vi "Affichage PokaenDex 1P.vi"() -> ()   [LabVIEW 2013]
uses:
  <vilib>/picture/picture.llb/Draw True-Color Pixmap.vi
panel:
  in  "Bouton OK 2":bool
  in  "Port USB en réception":refnum<visa-resource-name>="ASRL1::INSTR"
  out "Cache rouge":picture
  out "Image 2D":picture
  out "sign 1":u32
  out "Distance cible":string
  out "Cam D détect":bool
  out "2 cam détect":bool
  out "Cam G détect":bool
  in  "2D/3D":bool caption="Booléen 5"
  in  "Booléen":bool
  out "Ennemi":bool
  out "Ami":bool
  out "Cache gris":picture
  out "Nom du Pokaenmon":string
  out "Pokeanmon détécté !":bool
  in  "stop":bool
  out "Image Pokaenmon":picture
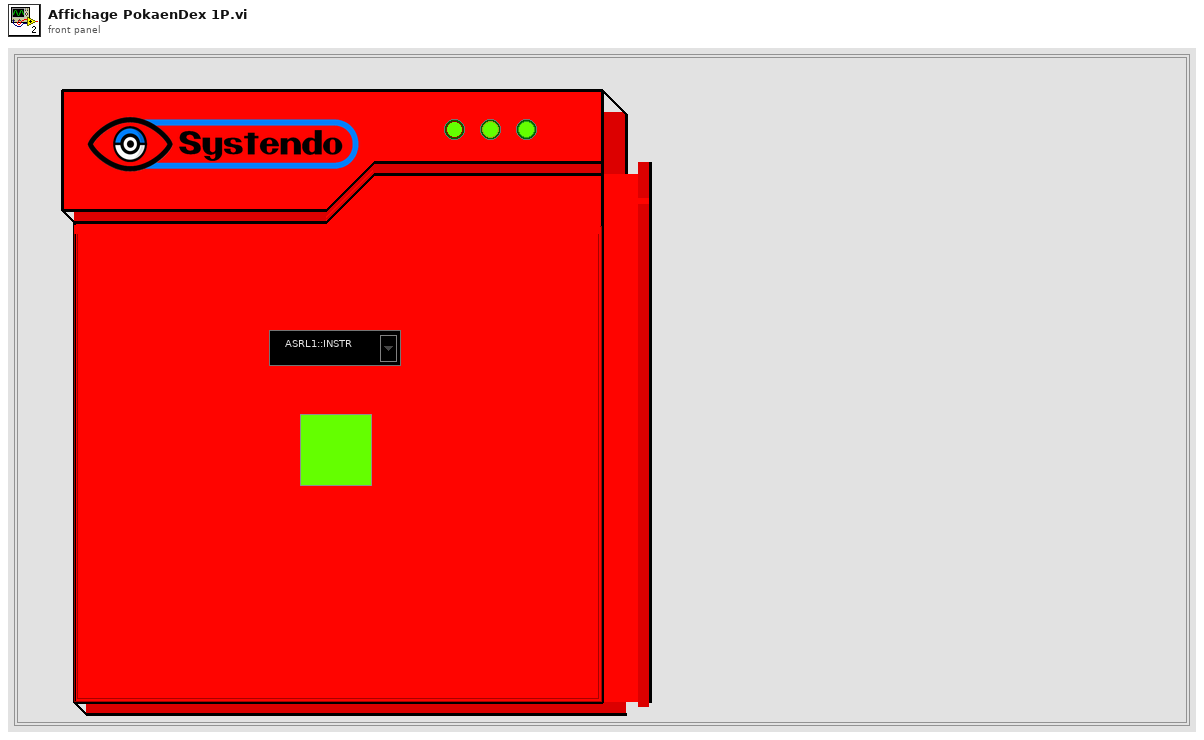
[diagram p1: front panel]
types:
  T1 = cluster{"Pokaenmon détecté":bool, "Signature":u32, "x":dbl, "y ":dbl, "Longueur":dbl, "Hauteur":dbl}
  T2 = cluster{"Données Caméra G":cluster{dbl, dbl, dbl, dbl}, "Données Caméra D":cluster{dbl, dbl, dbl, dbl}}
  T3 = typedef "imagedata.ctl" = cluster{"image type":i32, "image depth":i32, "image":u8[], "mask":u8[], "colors":u32[], "Rectangle":cluster{"left":i16, "top":i16, "right":i16, "bottom":i16}}
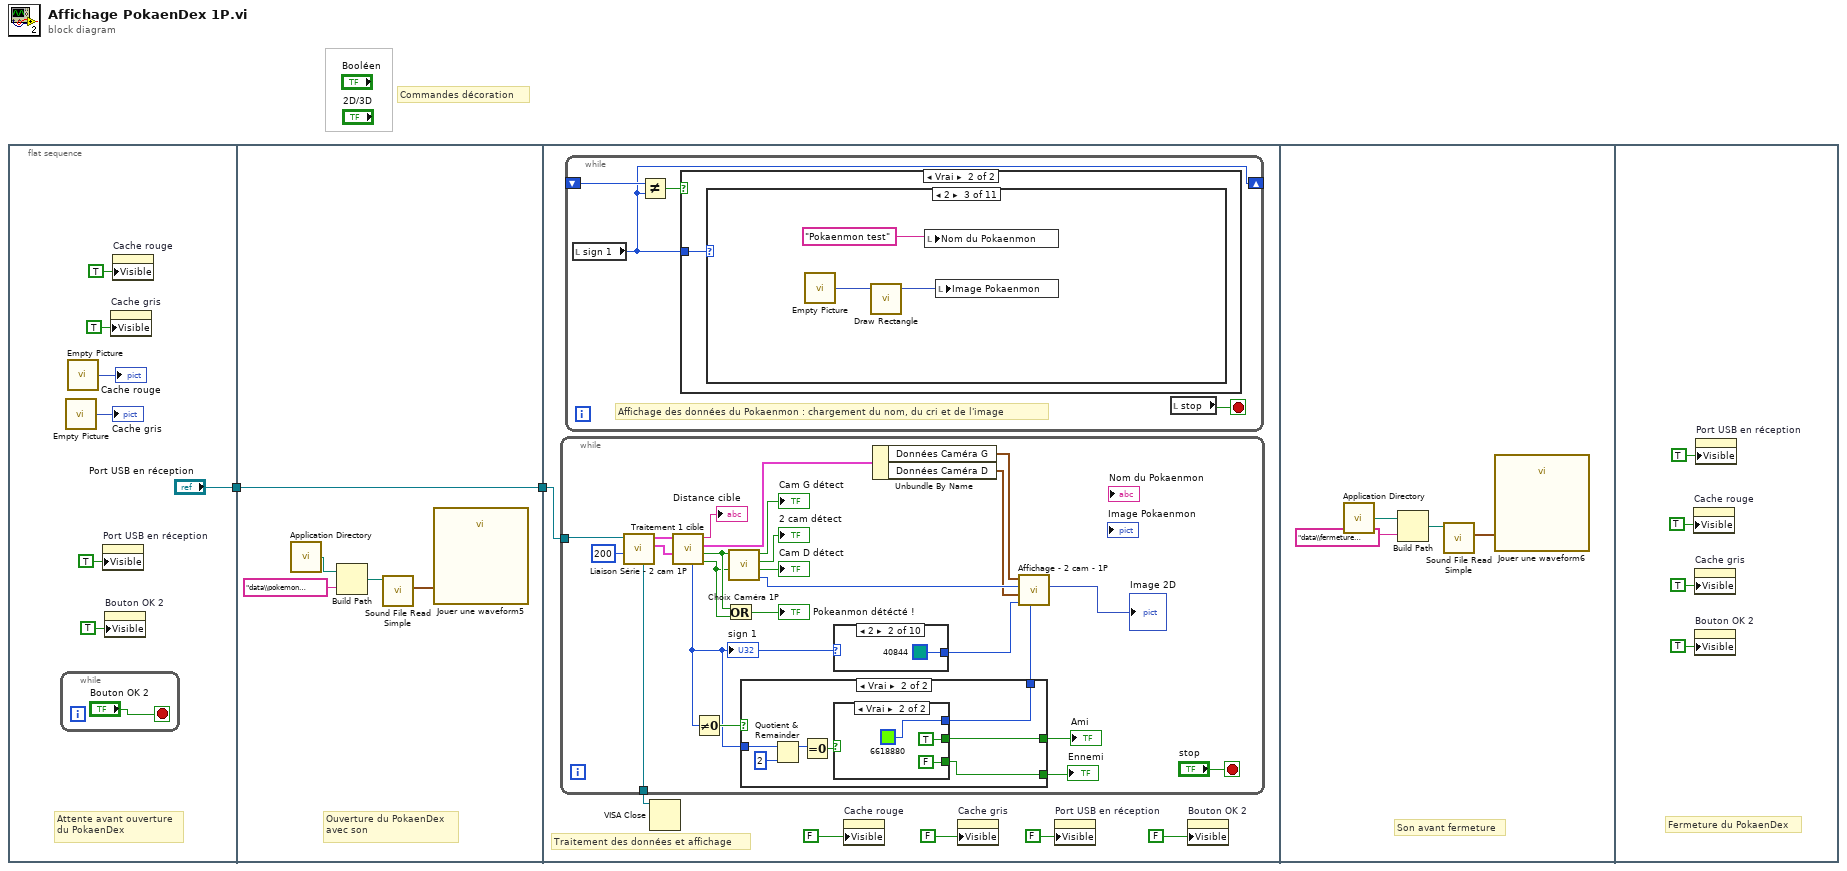
[diagram p0: block diagram]
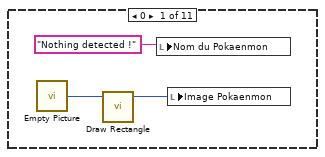
[diagram p3: hidden frame]
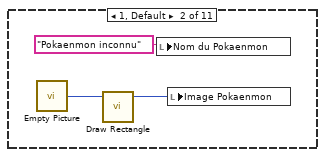
[diagram p4: hidden frame]
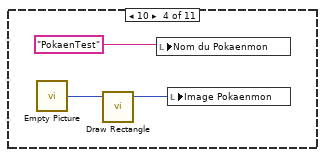
[diagram p5: hidden frame]
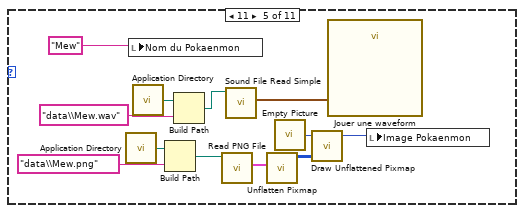
[diagram p6: hidden frame]
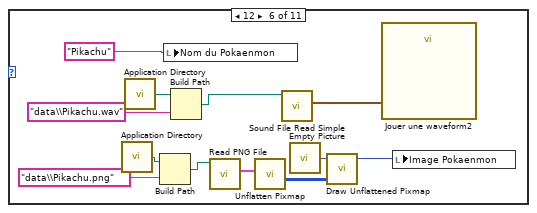
[diagram p7: hidden frame]
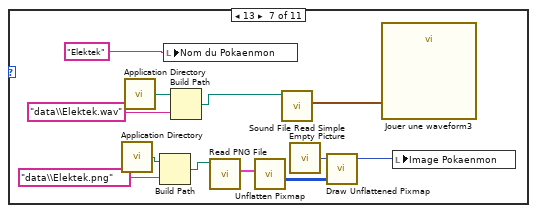
[diagram p8: hidden frame]
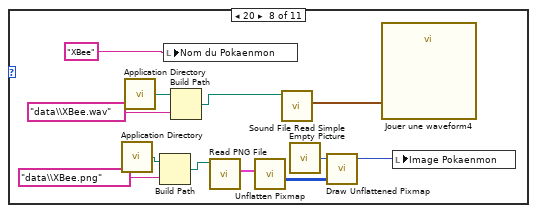
[diagram p9: hidden frame]
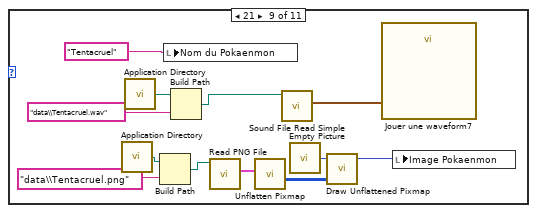
[diagram p10: hidden frame]
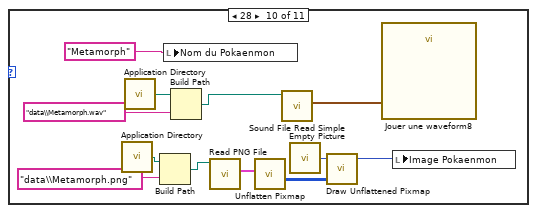
[diagram p11: hidden frame]
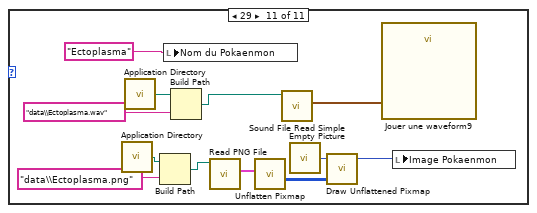
[diagram p12: hidden frame]
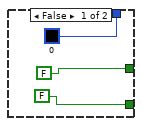
[diagram p13: hidden frame]
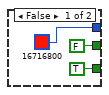
[diagram p14: hidden frame]
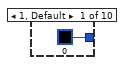
[diagram p15: hidden frame]
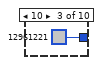
[diagram p16: hidden frame]
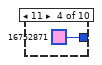
[diagram p17: hidden frame]
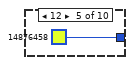
[diagram p18: hidden frame]
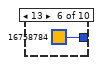
[diagram p19: hidden frame]
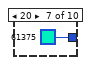
[diagram p20: hidden frame]
diagram:
  # "Commandes décoration"
  n1 = flat-sequence {
    tunnel: ["Port USB en réception"] -> w2
    tunnel: w2 -> [w15]
    tunnel: [w15] -> w1
    tunnel: w1 -> [w20]
    frame #0 {
      # "Attente avant ouverture\ndu PokaenDex"
      n2 = while {
        stop <- "Bouton OK 2" stop-if-true
      }
      n3 = call "Empty Picture"() -> ("empty picture"=→"Cache gris":picture)
      n4 = call "Empty Picture"() -> ("empty picture"=→"Cache rouge":picture)
      n5 = property on="Port USB en réception" class="NomVISA"("Visible"=TRUE) -> ()  [unwired: 2 in, 2 out]
      n6 = property on="Bouton OK 2" class="Bool"("Visible"=TRUE) -> ()  [unwired: 2 in, 2 out]
      n7 = property on="Cache gris" class="Image"("Visible"=TRUE) -> ()  [unwired: 2 in, 2 out]
      n8 = property on="Cache rouge" class="Image"("Visible"=TRUE) -> ()  [unwired: 2 in, 2 out]
    }
    frame #1 {
      # "Ouverture du PokaenDex\navec son"
      n9 = call <vilib>:"Application Directory.vi"() -> ("Application Directory"=w11:path)
      n10 = Build Path(base path=w11, name or relative path="data\\pokemon ouverture.wav") -> (appended path=w12:path)
      n11 = call <vilib>:"Sound File Read Simple.vi"("path"=w12) -> ("data"=w14:waveform(dbl)[])  [unwired: 7 in, 3 out]
      n12 = call "Jouer une waveform5"("Data"=w14) -> ()  [unwired: 18 in, 1 out]
    }
    frame #2 {
      # "Traitement des données et affichage"
      n13 = while {
        tunnel: w20 -> [w138]
        tunnel: [w137] -> w21
        stop <- "stop" stop-if-true
        n14 = call "Liaison Série - 2 cam 1P.vi"("timeout (ms)"=u32 200 ("timeout (10sec)"), "Port USB en réception"=w138) -> ("Indications pokaenmon D"=w130:T1, "Indications pokaenmon G"=w136:T1, "Nom VISA en sortie"=w137:refnum<visa-resource-name>)  [unwired: 7 in]
        n15 = call "Traitement 1 cible.vi"("Indications Pokaenmon D"=w130, "Indications Pokaenmon G"=w136) -> ("D détect"=w132:bool, "G détect"=w133:bool, "Données caméras"=w128:T2, "Distance"=→"Distance cible":string, "Signature"=w125:u32)  [unwired: 5 in]
        "sign 1" <- w125
        n16 = Not Equal To 0?(x=w125) -> (x != 0?=w126:bool)
        n17 = Or(x=w133, y=w132) -> (x .or. y?=→"Pokeanmon détécté !":bool)
        n18 = call "Choix Caméra 1P.vi"("Detecté caméra D"=w132, "Detecté caméra G"=w133) -> ("Choix"=w144:u16, "Detecté caméra D"=→"Cam D détect":bool, "Detecté caméra G et D"=→"2 cam détect":bool, "Detecté caméra G"=→"Cam G détect":bool)  [unwired: 6 in]
        n19 = case shown="Vrai" w126 {
          tunnel: w125 -> [_ w153]
          tunnel: [u32 0 ("Couleur rectangle") w152] -> w127
          tunnel: [FALSE w151] -> w124
          tunnel: [FALSE w150] -> w123
          frame False {
          }
          frame True {
            n20 = Quotient & Remainder(x=w153, y=2) -> (x-y*floor(x/y)=w155:u32)  [unwired: 1 out]
            n21 = Equal To 0?(x=w155) -> (x = 0?=w156:bool)
            n22 = case shown="Vrai" w156 {
              tunnel: [FALSE TRUE] -> w151
              tunnel: [TRUE FALSE] -> w150
              tunnel: [u32 16716800 ("Couleur rectangle") u32 6618880 ("Couleur rectangle")] -> w152
              frame False {
              }
              frame True {
              }
            }
          }
        }
        "Ami" <- w124
        "Ennemi" <- w123
        n23 = case shown="2" w125 {
          tunnel: [u32 0 ("Couleur rectangle") u32 40844 ("Couleur rectangle") u32 12961221 ("Couleur rectangle") u32 16752871 ("Couleur rectangle") u32 14876458 ("Couleur rectangle") u32 16758784 ("Couleur rectangle") u32 61375 ("Couleur rectangle") u32 6499071 ("Couleur rectangle") u32 15663254 ("Couleur rectangle") u32 10092783 ("Couleur rectangle")] -> w145
          frame 1, Default {
          }
          frame 2 {
          }
          frame 10 {
          }
          frame 11 {
          }
          frame 12 {
          }
          frame 13 {
          }
          frame 20 {
          }
          frame 21 {
          }
          frame 29 {
          }
          frame 28 {
          }
        }
        n24 = Unbundle By Name(w128) -> ("Données Caméra G"=w134:cluster{dbl, dbl, dbl, dbl}, "Données Caméra D"=w135:cluster{dbl, dbl, dbl, dbl})
        n25 = call "Affichage - 2 cam - 1P.vi"("Couleur fond"=w127, "Couleur rectangle"=w145, "Caméra D"=w135, "Choix cam"=w144, "Caméra G"=w134) -> ("Image 2D"=→"Image 2D":picture)  [unwired: 6 in]
      }
      n26 = while {
        shift-right: [w22] -> _
        shift-left: _ -> [w24]
        stop <- w25 stop-if-true
        # "Affichage des données du Pokaenmon : chargement du nom, du cri et de l'image"
        n27 = local read "sign 1"() -> (w22:u32)
        n28 = Not Equal?(x=w24, y=w22) -> (x != y?=w23:bool)
        n29 = case shown="Vrai" w23 {
          tunnel: w22 -> [_ w26]
          frame False {
          }
          frame True {
            n30 = case shown="2" w26 {
              frame 0 {
                n31 = call "Empty Picture"() -> ("empty picture"=w29:picture)
                n32 = call <vilib>:"Draw Rectangle.vi"("picture"=w29) -> ("new picture"=w27:picture)  [unwired: 8 in]
                n33 = local write "Nom du Pokaenmon"("Nothing detected !") -> ()
                n34 = local write "Image Pokaenmon"(w27) -> ()
              }
              frame 1, Default {
                n35 = call "Empty Picture"() -> ("empty picture"=w32:picture)
                n36 = call <vilib>:"Draw Rectangle.vi"("picture"=w32) -> ("new picture"=w30:picture)  [unwired: 8 in]
                n37 = local write "Nom du Pokaenmon"("Pokaenmon inconnu") -> ()
                n38 = local write "Image Pokaenmon"(w30) -> ()
              }
              frame 2 {
                n39 = call "Empty Picture"() -> ("empty picture"=w35:picture)
                n40 = call <vilib>:"Draw Rectangle.vi"("picture"=w35) -> ("new picture"=w33:picture)  [unwired: 8 in]
                n41 = local write "Nom du Pokaenmon"("Pokaenmon test") -> ()
                n42 = local write "Image Pokaenmon"(w33) -> ()
              }
              frame 10 {
                n43 = call "Empty Picture"() -> ("empty picture"=w38:picture)
                n44 = call <vilib>:"Draw Rectangle.vi"("picture"=w38) -> ("new picture"=w36:picture)  [unwired: 8 in]
                n45 = local write "Nom du Pokaenmon"("PokaenTest") -> ()
                n46 = local write "Image Pokaenmon"(w36) -> ()
              }
              frame 11 {
                n47 = call <vilib>:"Application Directory.vi"() -> ("Application Directory"=w39:path)
                n48 = local write "Nom du Pokaenmon"("Mew") -> ()
                n49 = call <vilib>:"Application Directory.vi"() -> ("Application Directory"=w40:path)
                n50 = Build Path(base path=w39, name or relative path="data\\Mew.png") -> (appended path=w41:path)
                n51 = Build Path(base path=w40, name or relative path="data\\Mew.wav") -> (appended path=w43:path)
                n52 = call <vilib>:"Read PNG File.vi"("path to PNG file"=w41) -> ("image data"=w49:T3)  [unwired: 8 in, 2 out]
                n53 = call <vilib>:"Sound File Read Simple.vi"("path"=w43) -> ("data"=w45:waveform(dbl)[])  [unwired: 7 in, 3 out]
                n54 = call <vilib>:"Unflatten Pixmap.vi"("image data"=w49) -> ("24-bit pixmap"=w48:u32[][])  [unwired: 4 in, 6 out]
                n55 = call "Empty Picture"() -> ("empty picture"=w50:picture)
                n56 = call-poly <vilib>:"Draw Unflattened Pixmap.vi"("picture"=w50, "data (RGB format)"=w48) -> ("new picture"=w46:picture)  [unwired: 7 in]
                n57 = call "Jouer une waveform"("Data"=w45) -> ()  [unwired: 18 in, 1 out]
                n58 = local write "Image Pokaenmon"(w46) -> ()
              }
              frame 12 {
                n59 = call <vilib>:"Application Directory.vi"() -> ("Application Directory"=w51:path)
                n60 = call <vilib>:"Application Directory.vi"() -> ("Application Directory"=w52:path)
                n61 = Build Path(base path=w51, name or relative path="data\\Pikachu.png") -> (appended path=w55:path)
                n62 = local write "Nom du Pokaenmon"("Pikachu") -> ()
                n63 = Build Path(base path=w52, name or relative path="data\\Pikachu.wav") -> (appended path=w53:path)
                n64 = call <vilib>:"Read PNG File.vi"("path to PNG file"=w55) -> ("image data"=w61:T3)  [unwired: 8 in, 2 out]
                n65 = call <vilib>:"Unflatten Pixmap.vi"("image data"=w61) -> ("24-bit pixmap"=w60:u32[][])  [unwired: 4 in, 6 out]
                n66 = call <vilib>:"Sound File Read Simple.vi"("path"=w53) -> ("data"=w57:waveform(dbl)[])  [unwired: 7 in, 3 out]
                n67 = call "Empty Picture"() -> ("empty picture"=w62:picture)
                n68 = call-poly <vilib>:"Draw Unflattened Pixmap.vi"("picture"=w62, "data (RGB format)"=w60) -> ("new picture"=w58:picture)  [unwired: 7 in]
                n69 = call "Jouer une waveform2"("Data"=w57) -> ()  [unwired: 18 in, 1 out]
                n70 = local write "Image Pokaenmon"(w58) -> ()
              }
              frame 13 {
                n71 = call <vilib>:"Application Directory.vi"() -> ("Application Directory"=w63:path)
                n72 = call <vilib>:"Application Directory.vi"() -> ("Application Directory"=w64:path)
                n73 = Build Path(base path=w63, name or relative path="data\\Elektek.png") -> (appended path=w67:path)
                n74 = local write "Nom du Pokaenmon"("Elektek") -> ()
                n75 = Build Path(base path=w64, name or relative path="data\\Elektek.wav") -> (appended path=w65:path)
                n76 = call <vilib>:"Read PNG File.vi"("path to PNG file"=w67) -> ("image data"=w73:T3)  [unwired: 8 in, 2 out]
                n77 = call <vilib>:"Unflatten Pixmap.vi"("image data"=w73) -> ("24-bit pixmap"=w72:u32[][])  [unwired: 4 in, 6 out]
                n78 = call <vilib>:"Sound File Read Simple.vi"("path"=w65) -> ("data"=w69:waveform(dbl)[])  [unwired: 7 in, 3 out]
                n79 = call "Empty Picture"() -> ("empty picture"=w74:picture)
                n80 = call-poly <vilib>:"Draw Unflattened Pixmap.vi"("picture"=w74, "data (RGB format)"=w72) -> ("new picture"=w70:picture)  [unwired: 7 in]
                n81 = call "Jouer une waveform3"("Data"=w69) -> ()  [unwired: 18 in, 1 out]
                n82 = local write "Image Pokaenmon"(w70) -> ()
              }
              frame 20 {
                n83 = call <vilib>:"Application Directory.vi"() -> ("Application Directory"=w75:path)
                n84 = call <vilib>:"Application Directory.vi"() -> ("Application Directory"=w76:path)
                n85 = Build Path(base path=w75, name or relative path="data\\XBee.png") -> (appended path=w79:path)
                n86 = local write "Nom du Pokaenmon"("XBee") -> ()
                n87 = Build Path(base path=w76, name or relative path="data\\XBee.wav") -> (appended path=w77:path)
                n88 = call <vilib>:"Read PNG File.vi"("path to PNG file"=w79) -> ("image data"=w85:T3)  [unwired: 8 in, 2 out]
                n89 = call <vilib>:"Unflatten Pixmap.vi"("image data"=w85) -> ("24-bit pixmap"=w84:u32[][])  [unwired: 4 in, 6 out]
                n90 = call <vilib>:"Sound File Read Simple.vi"("path"=w77) -> ("data"=w81:waveform(dbl)[])  [unwired: 7 in, 3 out]
                n91 = call "Empty Picture"() -> ("empty picture"=w86:picture)
                n92 = call-poly <vilib>:"Draw Unflattened Pixmap.vi"("picture"=w86, "data (RGB format)"=w84) -> ("new picture"=w82:picture)  [unwired: 7 in]
                n93 = call "Jouer une waveform4"("Data"=w81) -> ()  [unwired: 18 in, 1 out]
                n94 = local write "Image Pokaenmon"(w82) -> ()
              }
              frame 21 {
                n95 = call <vilib>:"Application Directory.vi"() -> ("Application Directory"=w87:path)
                n96 = call <vilib>:"Application Directory.vi"() -> ("Application Directory"=w88:path)
                n97 = Build Path(base path=w87, name or relative path="data\\Tentacruel.png") -> (appended path=w91:path)
                n98 = local write "Nom du Pokaenmon"("Tentacruel") -> ()
                n99 = Build Path(base path=w88, name or relative path="data\\Tentacruel.wav") -> (appended path=w89:path)
                n100 = call <vilib>:"Read PNG File.vi"("path to PNG file"=w91) -> ("image data"=w97:T3)  [unwired: 8 in, 2 out]
                n101 = call <vilib>:"Unflatten Pixmap.vi"("image data"=w97) -> ("24-bit pixmap"=w96:u32[][])  [unwired: 4 in, 6 out]
                n102 = call <vilib>:"Sound File Read Simple.vi"("path"=w89) -> ("data"=w93:waveform(dbl)[])  [unwired: 7 in, 3 out]
                n103 = call "Empty Picture"() -> ("empty picture"=w98:picture)
                n104 = call-poly <vilib>:"Draw Unflattened Pixmap.vi"("picture"=w98, "data (RGB format)"=w96) -> ("new picture"=w94:picture)  [unwired: 7 in]
                n105 = call "Jouer une waveform7"("Data"=w93) -> ()  [unwired: 18 in, 1 out]
                n106 = local write "Image Pokaenmon"(w94) -> ()
              }
              frame 28 {
                n107 = call <vilib>:"Application Directory.vi"() -> ("Application Directory"=w99:path)
                n108 = call <vilib>:"Application Directory.vi"() -> ("Application Directory"=w100:path)
                n109 = Build Path(base path=w99, name or relative path="data\\Metamorph.png") -> (appended path=w103:path)
                n110 = local write "Nom du Pokaenmon"("Metamorph") -> ()
                n111 = Build Path(base path=w100, name or relative path="data\\Metamorph.wav") -> (appended path=w101:path)
                n112 = call <vilib>:"Read PNG File.vi"("path to PNG file"=w103) -> ("image data"=w109:T3)  [unwired: 8 in, 2 out]
                n113 = call <vilib>:"Unflatten Pixmap.vi"("image data"=w109) -> ("24-bit pixmap"=w108:u32[][])  [unwired: 4 in, 6 out]
                n114 = call <vilib>:"Sound File Read Simple.vi"("path"=w101) -> ("data"=w105:waveform(dbl)[])  [unwired: 7 in, 3 out]
                n115 = call "Empty Picture"() -> ("empty picture"=w110:picture)
                n116 = call-poly <vilib>:"Draw Unflattened Pixmap.vi"("picture"=w110, "data (RGB format)"=w108) -> ("new picture"=w106:picture)  [unwired: 7 in]
                n117 = call "Jouer une waveform8"("Data"=w105) -> ()  [unwired: 18 in, 1 out]
                n118 = local write "Image Pokaenmon"(w106) -> ()
              }
              frame 29 {
                n119 = call <vilib>:"Application Directory.vi"() -> ("Application Directory"=w111:path)
                n120 = call <vilib>:"Application Directory.vi"() -> ("Application Directory"=w112:path)
                n121 = Build Path(base path=w111, name or relative path="data\\Ectoplasma.png") -> (appended path=w115:path)
                n122 = local write "Nom du Pokaenmon"("Ectoplasma") -> ()
                n123 = Build Path(base path=w112, name or relative path="data\\Ectoplasma.wav") -> (appended path=w113:path)
                n124 = call <vilib>:"Read PNG File.vi"("path to PNG file"=w115) -> ("image data"=w121:T3)  [unwired: 8 in, 2 out]
                n125 = call <vilib>:"Unflatten Pixmap.vi"("image data"=w121) -> ("24-bit pixmap"=w120:u32[][])  [unwired: 4 in, 6 out]
                n126 = call <vilib>:"Sound File Read Simple.vi"("path"=w113) -> ("data"=w117:waveform(dbl)[])  [unwired: 7 in, 3 out]
                n127 = call "Empty Picture"() -> ("empty picture"=w122:picture)
                n128 = call-poly <vilib>:"Draw Unflattened Pixmap.vi"("picture"=w122, "data (RGB format)"=w120) -> ("new picture"=w118:picture)  [unwired: 7 in]
                n129 = call "Jouer une waveform9"("Data"=w117) -> ()  [unwired: 18 in, 1 out]
                n130 = local write "Image Pokaenmon"(w118) -> ()
              }
            }
          }
        }
        n131 = local read "stop"() -> (w25:bool)
      }
      n132 = VISA Close(VISA resource name=w21) -> ()  [unwired: 1 in, 1 out]
      n133 = property on="Cache rouge" class="Image"("Visible"=FALSE) -> ()  [unwired: 2 in, 2 out]
      n134 = property on="Cache gris" class="Image"("Visible"=FALSE) -> ()  [unwired: 2 in, 2 out]
      n135 = property on="Port USB en réception" class="NomVISA"("Visible"=FALSE) -> ()  [unwired: 2 in, 2 out]
      n136 = property on="Bouton OK 2" class="Bool"("Visible"=FALSE) -> ()  [unwired: 2 in, 2 out]
    }
    frame #3 {
      # "Son avant fermeture"
      n137 = call <vilib>:"Application Directory.vi"() -> ("Application Directory"=w173:path)
      n138 = Build Path(base path=w173, name or relative path="data\\fermeture pokedex.wav") -> (appended path=w174:path)
      n139 = call <vilib>:"Sound File Read Simple.vi"("path"=w174) -> ("data"=w176:waveform(dbl)[])  [unwired: 7 in, 3 out]
      n140 = call "Jouer une waveform6"("Data"=w176) -> ()  [unwired: 18 in, 1 out]
    }
    frame #4 {
      # "Fermeture du PokaenDex"
      n141 = property on="Cache rouge" class="Image"("Visible"=TRUE) -> ()  [unwired: 2 in, 2 out]
      n142 = property on="Cache gris" class="Image"("Visible"=TRUE) -> ()  [unwired: 2 in, 2 out]
      n143 = property on="Bouton OK 2" class="Bool"("Visible"=TRUE) -> ()  [unwired: 2 in, 2 out]
      n144 = property on="Port USB en réception" class="NomVISA"("Visible"=TRUE) -> ()  [unwired: 2 in, 2 out]
    }
  }
